vi "TAT_Time Lock.vi"(8 "error in":errorcluster) -> (0 "error out":errorcluster, 3 "Time Laps or MAC ?":bool)   [LabVIEW 2017]
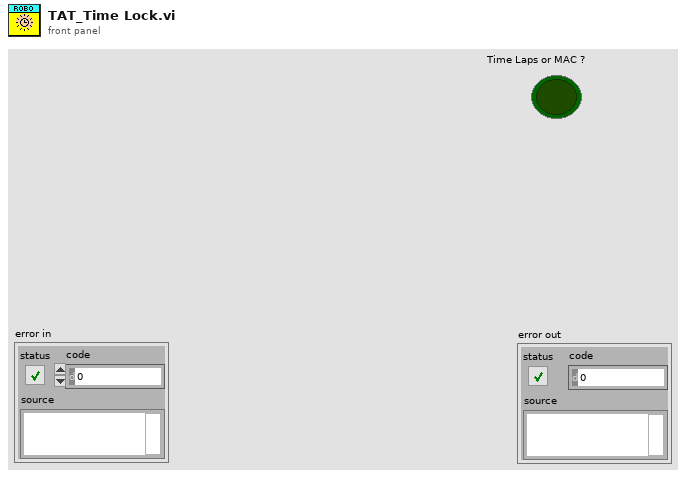
[diagram p1: front panel]
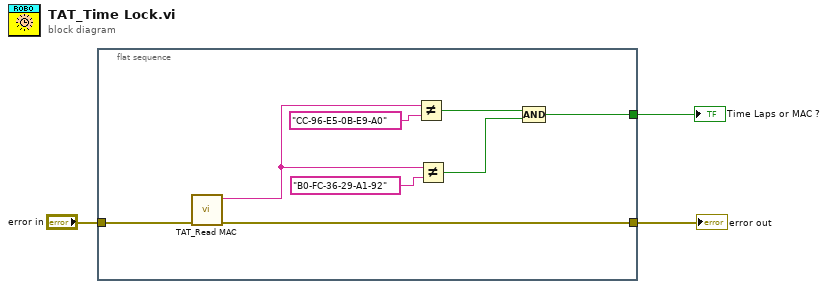
[diagram p0: block diagram]
diagram:
  n1 = flat-sequence {
    tunnel: [w4] -> w2
    tunnel: "error in" -> [w11]
    tunnel: [w10] -> w1
    frame #0 {
      n2 = call "TAT_Read MAC.vi"("error in (no error)"=w11) -> ("error out"=w10:errorcluster, "MAC1"=w9:string)  [unwired: 8 in, 1 out]
      n3 = Not Equal?(x=w9, y="CC-96-E5-0B-E9-A0") -> (x != y?=w5:bool)
      n4 = Not Equal?(x=w9, y="B0-FC-36-29-A1-92") -> (x != y?=w8:bool)
      n5 = Compound Arithmetic op=AND(w5, w8) -> (w4:bool)
    }
  }
  "Time Laps or MAC ?" <- w2
  "error out" <- w1
